vi "Global_1.vi"() -> ()   [LabVIEW 2016]
panel:
  in  "Stop Button_1":bool
  out "Numeric Control_1":dbl
  out "Boolean_1":bool
  out "Comunicacion_1":string
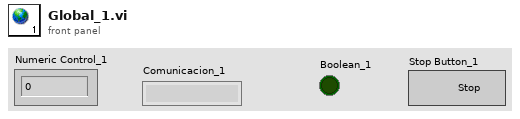
[diagram p1: front panel]
diagram:
